vi "Read Lockin Digitizer Configuration.vi"(8 "error in (no error)":errorcluster, 11 "DAQmx DAQmx Digitizer in":refnum<class "DAQmx Digitizer.lvclass">) -> (0 "error out":errorcluster, 2 "Configuration":T1={"Post-trigger delay"=0.01, "Post-trigger duration"=0.1, "Rate"=1000000.0, "Ranges"=[10.0], "Re-name channels"=[], "Active channels"="0:1", "External\nclock"=FALSE, "Frequencies"=[], "Monitor time\nconstant"=1.0, "Output \namplitudes"=[], "Input\nchannles"=[], "Sync"=FALSE, "Lock-in input channel phases"=[]} {"Output \namplitudes" format="%#_6pV"; "Monitor time\nconstant" format="%#_6ps"; "Frequencies" format="%#_6pHz"; "Rate" format="%#_8pHz"; "Post-trigger duration" format="%#_6ps"; "Post-trigger delay" format="%#_6ps"; "Ranges" format="%#_6pV"}, 3 "DAQmx DAQmx Digitizer in":refnum<class "DAQmx Digitizer.lvclass">)   [LabVIEW 2021, in "DAQmx Digitizer.lvclass"]
uses:
  DAQmx Digitizer.lvclass
  C:/GitHub/NHMFL_Core/Libraries/Instruments/Instrument Driver/Instrument Driver.lvclass
  Instruments/Pulse Driver/Lockin Digitizer Driver/Lockin Digitizer Configuration.ctl
  DAQmx Digitizer.lvclass/DAQmx Digitizer.ctl
panel:
  # "Pulse config"
  # "Lock-in config"
  # "#0\n\n#1"
  # "Monitor config"
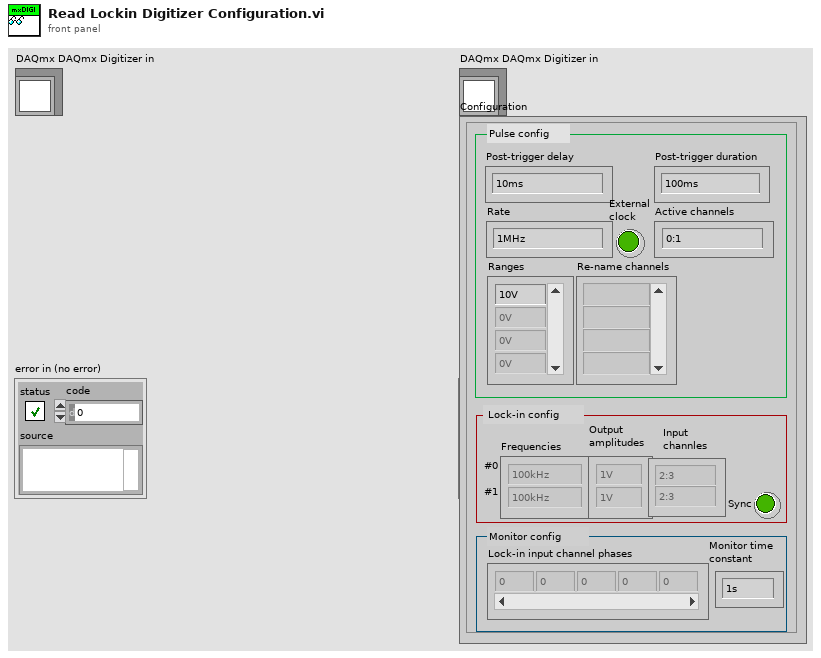
[diagram p1: front panel]
types:
  T1 = typedef "Lockin Digitizer Configuration.ctl" = cluster{"Post-trigger delay":dbl, "Post-trigger duration":dbl, "Rate":dbl, "Ranges":dbl[], "Re-name channels":string[], "Active channels":string, "External\nclock":bool, "Frequencies":dbl[], "Monitor time\nconstant":dbl, "Output \namplitudes":dbl[], "Input\nchannles":string[], "Sync":bool, "Lock-in input channel phases":dbl[]}
  T2 = typedef "Pusle Driver Configuration.ctl" = cluster{"Post-trigger delay":dbl, "Post-trigger duration":dbl, "Rate":dbl, "Ranges":dbl[], "Re-name channels":string[], "Active channels":string, "External clock":bool}
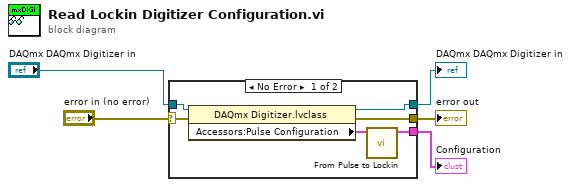
[diagram p0: block diagram]
diagram:
  n1 = case shown="No Error" "error in (no error)" {
    selector: "error in (no error)" -> [w11 w13]
    tunnel: [w6 w13] -> w2
    tunnel: [w9 w12] -> w1
    tunnel: "DAQmx DAQmx Digitizer in" -> [w8 w12]
    tunnel: [w10 _] -> w3
    frame No Error {
      n2 = property class="DAQmx Digitizer.lvclass"(reference=w8, error in=w11) -> (reference out=w9:refnum<class "DAQmx Digitizer.lvclass">, error out=w6:errorcluster, "Accessors:Pulse Configuration"=w7:T2)
      n3 = call "From Pulse to Lockin.vi"("Pulse Configuration in"=w7) -> ("Lockin Configuration out"=w10:T1)  [unwired: 10 in]
    }
    frame Error {
    }
  }
  "error out" <- w2
  "DAQmx DAQmx Digitizer in" <- w1
  "Configuration" <- w3
